vi "LinSpace (x0-dx-npts).vi"(3 "npts":i32=100, 4 "dx":dbl=1.0, 5 "x0":dbl) -> (0 "error out":errorcluster, 1 "Array":dbl[](array[numeric]))   [LabVIEW 2020]
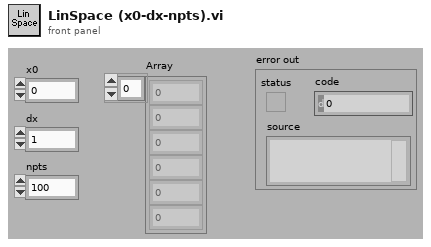
[diagram p1: front panel]
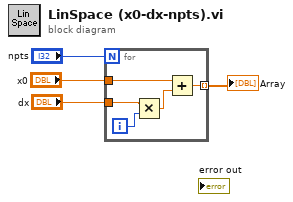
[diagram p0: block diagram]
diagram:
  n1 = for {
    N: "npts" -> [_]
    tunnel: "x0" -> [w6]
    tunnel: "dx" -> [w8]
    tunnel: [w5] -> w1 mode=indexing
    i -> [w9]
    n2 = Multiply(x=w8, y=w9) -> (x*y=w7:dbl)
    n3 = Add(x=w6, y=w7) -> (x+y=w5:dbl)
  }
  "Array" <- w1
